vi "test_ClientFGV_GetClientWithDifferentClusterId_Errors.vi"(8 "error in":errorcluster) -> (0 "error out":errorcluster, 2 "result":string, 3 "pass":bool)   [LabVIEW 2021, in "MeasurementServerTests.lvlib" / "Discovery Tests.lvlib"]
uses:
  Discovery Tests.lvlib
  Runtime/Clients/Discovery V1/TypeDefs/gRPC Client Cache FGV Action.ctl
  Fake Client Id Generator Action.ctl
  Runtime/Clients/Discovery V1/NI Discovery V1 Client.lvlib
  MeasurementServerTests.lvlib
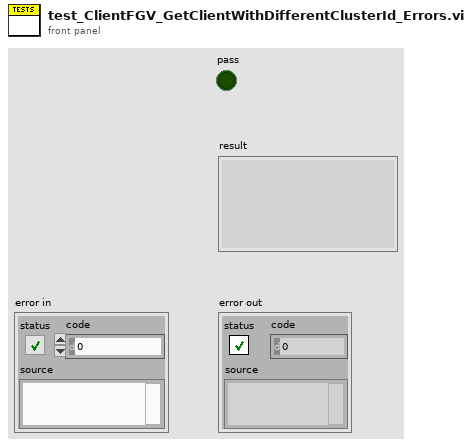
[diagram p1: front panel]
types:
  T1 = typedef "MeasurementServerTests.lvlib/Discovery Tests.lvlib/Fake Client Id Generator Action.ctl" = enum16{"Generate New Id", "Reset", "Error on Next Call"}
  T2 = typedef "NI Discovery V1 Client.lvlib/gRPC Client Cache FGV Action.ctl" = enum16{"Get Client", "Recreate Client", "Destroy Client", "Update ClusterId"}
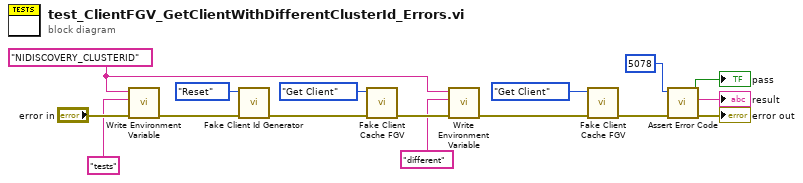
[diagram p0: block diagram]
diagram:
  w6 = "NIDISCOVERY_CLUSTERID" ("name")
  n1 = call "Write Environment Variable.vi"("error in"="error in", "value"="tests", "name"=w6) -> ("error out"=w11:errorcluster)  [unwired: 8 in]
  n2 = call "Fake Client Id Generator.vi"("error in"=w11, "action"=Fake_Client_Id_Generator_Action."Reset") -> ("error out"=w14:errorcluster)  [unwired: 8 in, 1 out]
  n3 = call "Fake Client Cache FGV.vi"("error in"=w14, "action"=gRPC_Client_Cache_FGV_Action."Get Client") -> ("error out"=w9:errorcluster)  [unwired: 7 in, 2 out]
  n4 = call "Write Environment Variable.vi"("error in"=w9, "value"="different", "name"=w6) -> ("error out"=w8:errorcluster)  [unwired: 8 in]
  n5 = call "Fake Client Cache FGV.vi"("error in"=w8, "action"=gRPC_Client_Cache_FGV_Action."Get Client") -> ("error out"=w5:errorcluster)  [unwired: 7 in, 2 out]
  n6 = call "Assert Error Code.vi"("error in"=w5, "expected error code"=5078) -> ("error out"=→"error out":errorcluster, "details"=→"result":string, "error code match?"=→"pass":bool)  [unwired: 7 in]
